vi "Add.vi"(1 "y":dbl, 2 "x":dbl) -> (0 "sum":dbl)   [LabVIEW 2014]
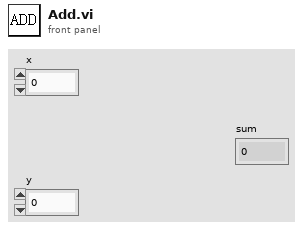
[diagram p1: front panel]
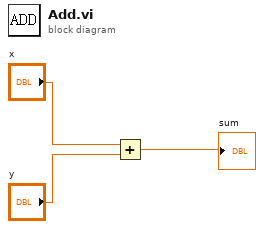
[diagram p0: block diagram]
diagram:
  n1 = Add(x="x", y="y") -> (x+y=→"sum":dbl)
